vi "prepAI_sealtest.vi"(2 "samples per channel":i32=1000) -> ()   [LabVIEW 2015]
uses:
  <vilib>/DAQmx/create/channels.llb/DAQmx Create Channel (AI-Voltage-Basic).vi
  <vilib>/DAQmx/configure/timing.llb/DAQmx Timing (Sample Clock).vi
panel:
  out "Terminal Name with Device Prefix":tag
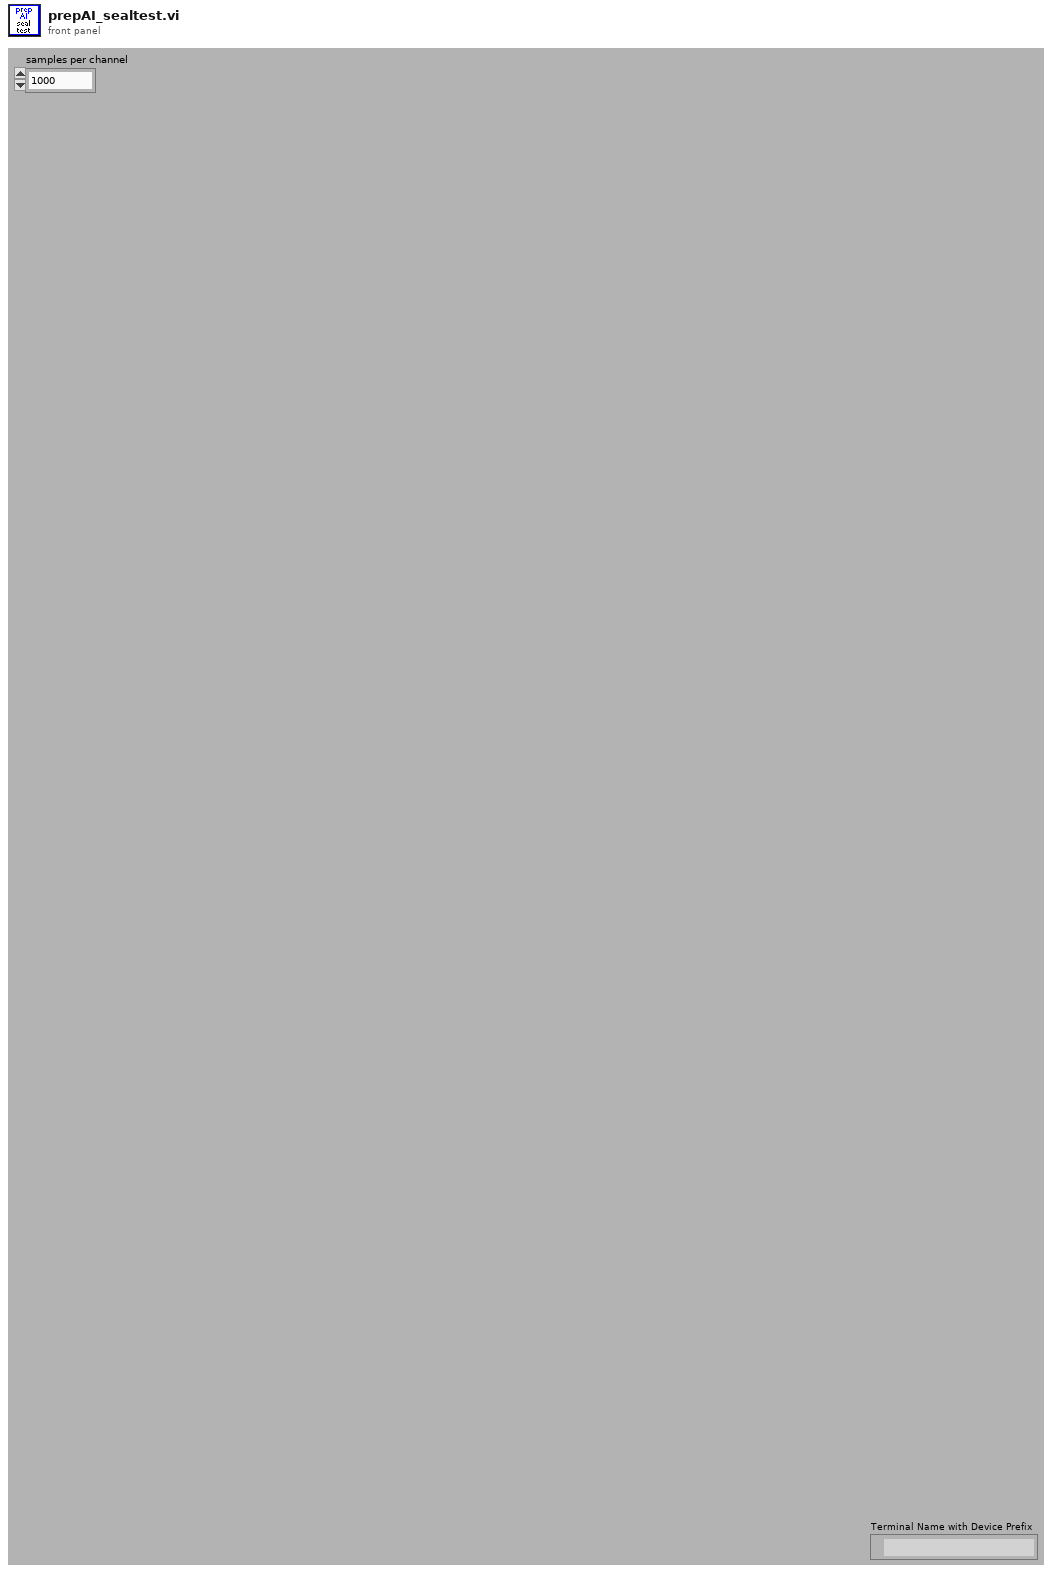
[diagram p1: front panel]
types:
  T1 = typedef "XYZStage.lvlib/XYZStage Configuration.ctl" = cluster{"VISA resource name":refnum<visa-resource-name>, "Timeout (3sec)":u32}
  T2 = cluster{"StageS":i32, "StageL":i32, "currmeas data dir":path, "image OD":u16, "contour OD":u16, "point OD":u16, "AOlines":tag[], "AIlines":tag[], "CI lines":tag[], "DO lines":tag[], "AO names":string[], "CI names":string[], "AI names":string[], "DO names":string[], "CIextensions":string[], "AIextensions":string[], "Voltage to Ygalvo":i32, "Voltage to Xgalvo":i32, "Voltage to patch":i32, "640 shutter":i32, "2P shutter":i32, "LT timestamp":u32, "Vp":i32, "Ip":i32, "camera trigger":i32, "master data dir":path, "voltage to Zpos":i32, "Vto2P":i32, "640 AO":i32, "488 AO":i32, "532 AO":i32, "640TTL":u32, "488TTL":u32, "532TTL":u32, "Device 1 sampleclock out":tag, "Device 1 Starttrigger out":tag, "Device 2 sampleclock in":tag, "Device 2 StartTrigger in ":tag, "2PODTTL":u32, "488 shutter":u32, "LCVR red":u32, "LCVR blue":u32, "Sutter Stage Config":T1}
  T3 = cluster{"AO parameters":cluster{"AOtab":dbl, "Repeats":dbl, "Cycles":dbl, "Start amplitude (V)":dbl, "Baseline (V)":dbl, "Step size (V)":dbl, "DC (%)":dbl, "Sampling frequency (Hz)":dbl, "Period (ms)":dbl, "Offset (V)":dbl, "Amplitude (V)":dbl, "Frequency":dbl, "Tri Repeats":dbl, "Cycle length (s)":dbl, "Pulses":dbl, "Matlab wave file":path, "Tri phase":dbl, "padding value":dbl}[]}
  T4 = cluster{"AOtab":dbl, "Repeats":dbl, "Cycles":dbl, "Start amplitude (V)":dbl, "Baseline (V)":dbl, "Step size (V)":dbl, "DC (%)":dbl, "Sampling frequency (Hz)":dbl, "Period (ms)":dbl, "Offset (V)":dbl, "Amplitude (V)":dbl, "Frequency":dbl, "Tri Repeats":dbl, "Cycle length (s)":dbl, "Pulses":dbl, "Matlab wave file":path, "Tri phase":dbl, "padding value":dbl}[]
  T5 = cluster{"AOtab":dbl, "Repeats":dbl, "Cycles":dbl, "Start amplitude (V)":dbl, "Baseline (V)":dbl, "Step size (V)":dbl, "DC (%)":dbl, "Sampling frequency (Hz)":dbl, "Period (ms)":dbl, "Offset (V)":dbl, "Amplitude (V)":dbl, "Frequency":dbl, "Tri Repeats":dbl, "Cycle length (s)":dbl, "Pulses":dbl, "Matlab wave file":path, "Tri phase":dbl, "padding value":dbl}
  T6 = cluster{" AI":refnum<k21>, "E_AI":errorcluster, "header":dbl[]}
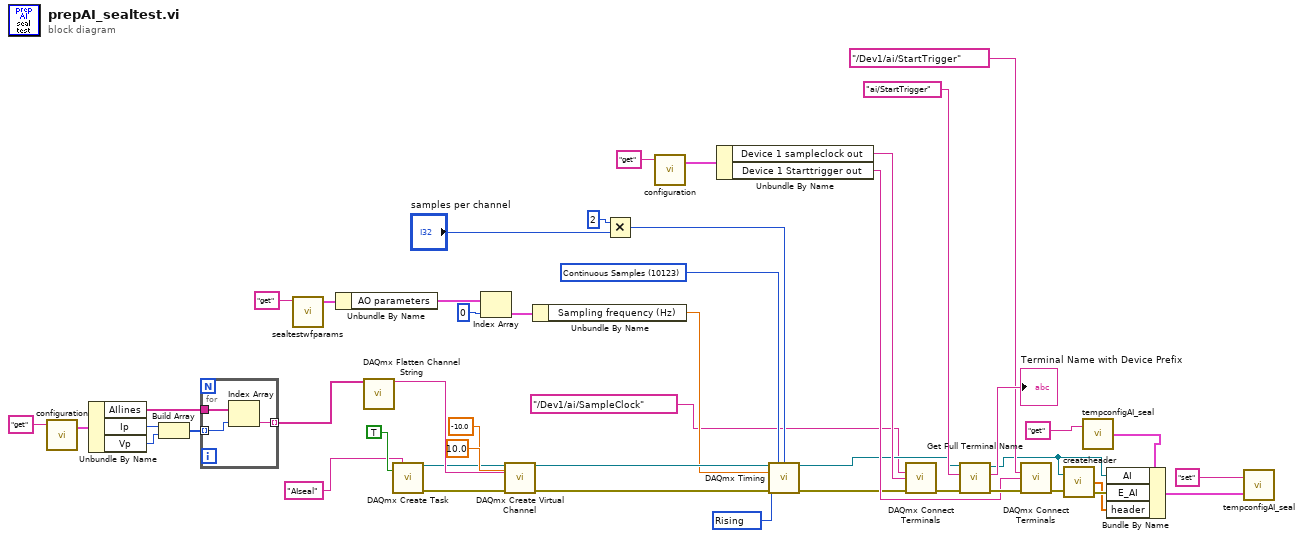
[diagram p0: block diagram]
diagram:
  w6 = 10280 items=["Rising"=10280, "Falling"=10171] ("active edge")
  w21 = 10123 items=["Finite Samples"=10178, "Continuous Samples"=10123, "Hardware Timed Single Point"=12522] ("sample mode")
  n1 = call "configuration.vi"("command"="get") -> ("config out"=w46:T2)  [unwired: 2 in, 1 out]
  n2 = Unbundle By Name(w46) -> ("AIlines"=w45:tag[], "Ip"=w41:i32, "Vp"=w42:i32)
  n3 = Build Array(w41, w42) -> (w40:i32[])
  n4 = for {
    tunnel: w40 -> [w50] mode=indexing
    tunnel: w45 -> [w49]
    tunnel: [w48] -> w44 mode=indexing
    n5 = Index Array(array=w49, index=w50) -> (element=w48:tag)
  }
  n6 = call "sealtestwfparams.vi"("command"="get") -> ("Params out"=w26:T3)  [unwired: 6 in]
  n7 = Unbundle By Name(w26) -> ("AO parameters"=w23:T4)
  n8 = call <vilib>:"DAQmx Flatten Channel String.vi"("names in"=w44) -> ("names out"=w43:string)  [unwired: 13 in, 1 out]
  n9 = call <vilib>:"DAQmx Create Task.vi"("new task name"="AIseal", "auto cleanup"=TRUE) -> ("task out"=w31:refnum<k21>, "error out"=w32:errorcluster)  [unwired: 12 in]
  n10 = Index Array(array=w23, index=0) -> (element=w24:T5)
  n11 = call-poly <vilib>:"DAQmx Create Virtual Channel.vi"("task in"=w31, "maximum value"=10.0, "minimum value"=-10.0, "physical channels"=w43, "error in"=w32) -> ("task out"=w39:refnum<k21>, "error out"=w38:errorcluster)  [unwired: 9 in]
  n12 = Unbundle By Name(w24) -> ("Sampling frequency (Hz)"=w20:dbl)
  n13 = Multiply(x=2, y="samples per channel") -> (x*y=w28:i32)
  n14 = call "configuration.vi"("command"="get") -> ("config out"=w14:T2)  [unwired: 2 in, 1 out]
  n15 = Unbundle By Name(w14) -> ("Device 1 sampleclock out"=w12:tag, "Device 1 Starttrigger out"=w11:tag)
  n16 = call-poly <vilib>:"DAQmx Timing.vi"("task/channels in"=w39, "sample mode"=w21, "samples per channel"=w28, "rate"=w20, "active edge"=w6, "error in"=w38) -> ("task out"=w10:refnum<k21>, "error out"=w8:errorcluster)  [unwired: 8 in]
  n17 = call <vilib>:"DAQmx Connect Terminals.vi"("source terminal"=tag "/Dev1/ai/SampleClock" ("source"), "destination terminal"=w12, "error in"=w8) -> ("error out"=w17:errorcluster)  [unwired: 12 in]
  n18 = call "Get Full Terminal Name.vi"("error in"=w17, "Local Terminal Name"="ai/StartTrigger", "task/channels in"=w10) -> ("error out"=w15:errorcluster, "Terminal Name with Device Prefix"=→"Terminal Name with Device Prefix":tag, "task out"=w9:refnum<k21>)  [unwired: 6 in]
  n19 = call <vilib>:"DAQmx Connect Terminals.vi"("source terminal"=tag "/Dev1/ai/StartTrigger", "destination terminal"=w11, "error in"=w15) -> ("error out"=w7:errorcluster)  [unwired: 12 in]
  n20 = call "createheader.vi"("task in"=w9, "error in"=w7) -> ("Array"=w34:dbl[], "error out"=w35:errorcluster)  [unwired: 1 out]
  n21 = call "tempconfigAI_seal.vi"("command"="get") -> ("Temp Config out"=w3:T6)  [unwired: 1 in]
  n22 = Bundle By Name(cluster=w3, "AI"=w9, "E_AI"=w35, "header"=w34) -> (w2:T6)
  n23 = call "tempconfigAI_seal.vi"("Temp Config in"=w2, "command"="set") -> ()  [unwired: 1 out]
